vi "Read Lookup Table.vi"(11 "TopicLookupTable in":refnum<class "TopicLookupTable.lvclass">) -> (2 "Topic Table":variant)   [LabVIEW 2015, in "Mediator.lvlib" / "TopicLookupTable.lvclass"]
doc: "<License>\nCopyright © 2017 Composed Systems, LLC | All rights reserved\nwww.composed.io\n\nAuthor: Ethan Stern <ethan.stern@composed.io>\n\nThis software is provided \"AS IS\" WITHOUT WARRANTIES, either express or implied, AND IS FOR EDUCATIONAL PURPOSES ONLY.\n</License>"
uses:
  TopicLookupTable.lvclass
  TopicLookupTable.lvclass/TopicLookupTable.ctl
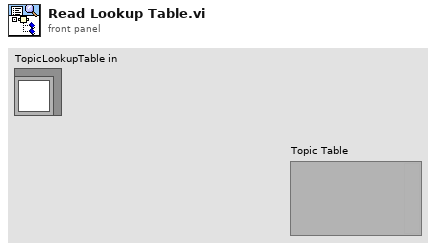
[diagram p1: front panel]
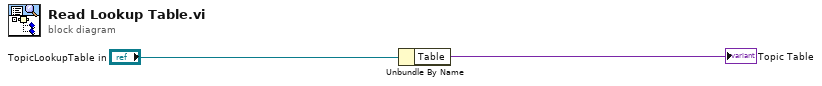
[diagram p0: block diagram]
diagram:
  n1 = Unbundle By Name("TopicLookupTable in") -> ("Table"=→"Topic Table":variant)
